vi "E_TO_DATA.vi"(10 "INPUT":string) -> (1 "子字符串":string, 2 "F-格式字符串":string)   [LabVIEW 2018]
panel:
  out "x*y":dbl
  out "数字":dbl
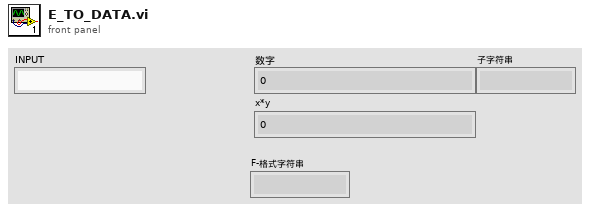
[diagram p1: front panel]
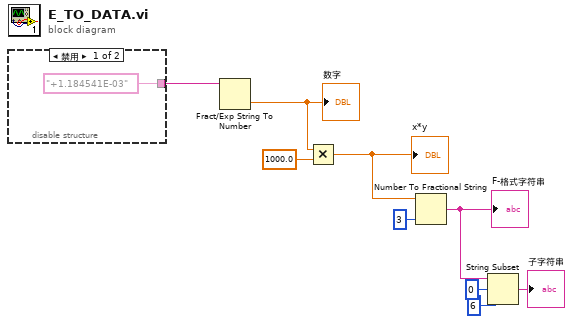
[diagram p0: block diagram]
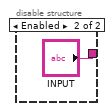
[diagram p2: hidden frame]
diagram:
  n1 = disable-structure shown="禁用" {
    disable-tunnel: ["+1.184541E-03" "INPUT"] -> w9
    frame Disabled {
    }
    frame Enabled {
    }
  }
  n2 = Fract/Exp String To Number(string=w9) -> (number=w8:dbl)  [unwired: 3 in, 1 out]
  "数字" <- w8
  n3 = Multiply(x=w8, y=1000.0) -> (x*y=w6:dbl)
  "x*y" <- w6
  n4 = Number To Fractional String(number=w6, precision (6)=i16 3 ("精度(6)")) -> (F-format string=w2:string)  [unwired: 2 in]
  "F-格式字符串" <- w2
  n5 = String Subset(string=w2, offset (0)=0 ("偏移量(0)"), length (rest)=6 ("长度（剩余）")) -> (substring=→"子字符串":string)
